vi "executeBuildSpecs.vi"() -> ()   [LabVIEW 2023]
doc: "Execute Build Specs G-CLI.vi\n----------------------------------------------\nThis VI is used to build the lvlibp from the build specifications.\n\nInputs:\n---------------------\n\n\nOutputs:\n---------------------\n\n\n----------------------------------------------\n1/27/2021 nina\nZühlke Engineering AG\nCH-8952 Schlieren\nwww.zuehlke.com"
uses:
  <vilib>/AppBuilder/AB_API_Simple/Get Build Specification Version (path).vi
  <vilib>/Wiresmith Technology/G CLI/CLI Class/CLI.lvclass
  <vilib>/AppBuilder/AB_API_Simple/NI_App_Builder_API.lvlib
panel:
  out "error out":errorcluster
  out "Build Specification Names":string[](array[string])
  # "Locals"
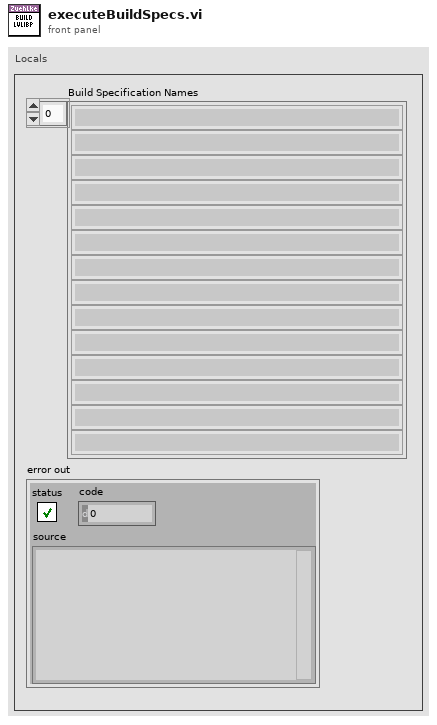
[diagram p1: front panel]
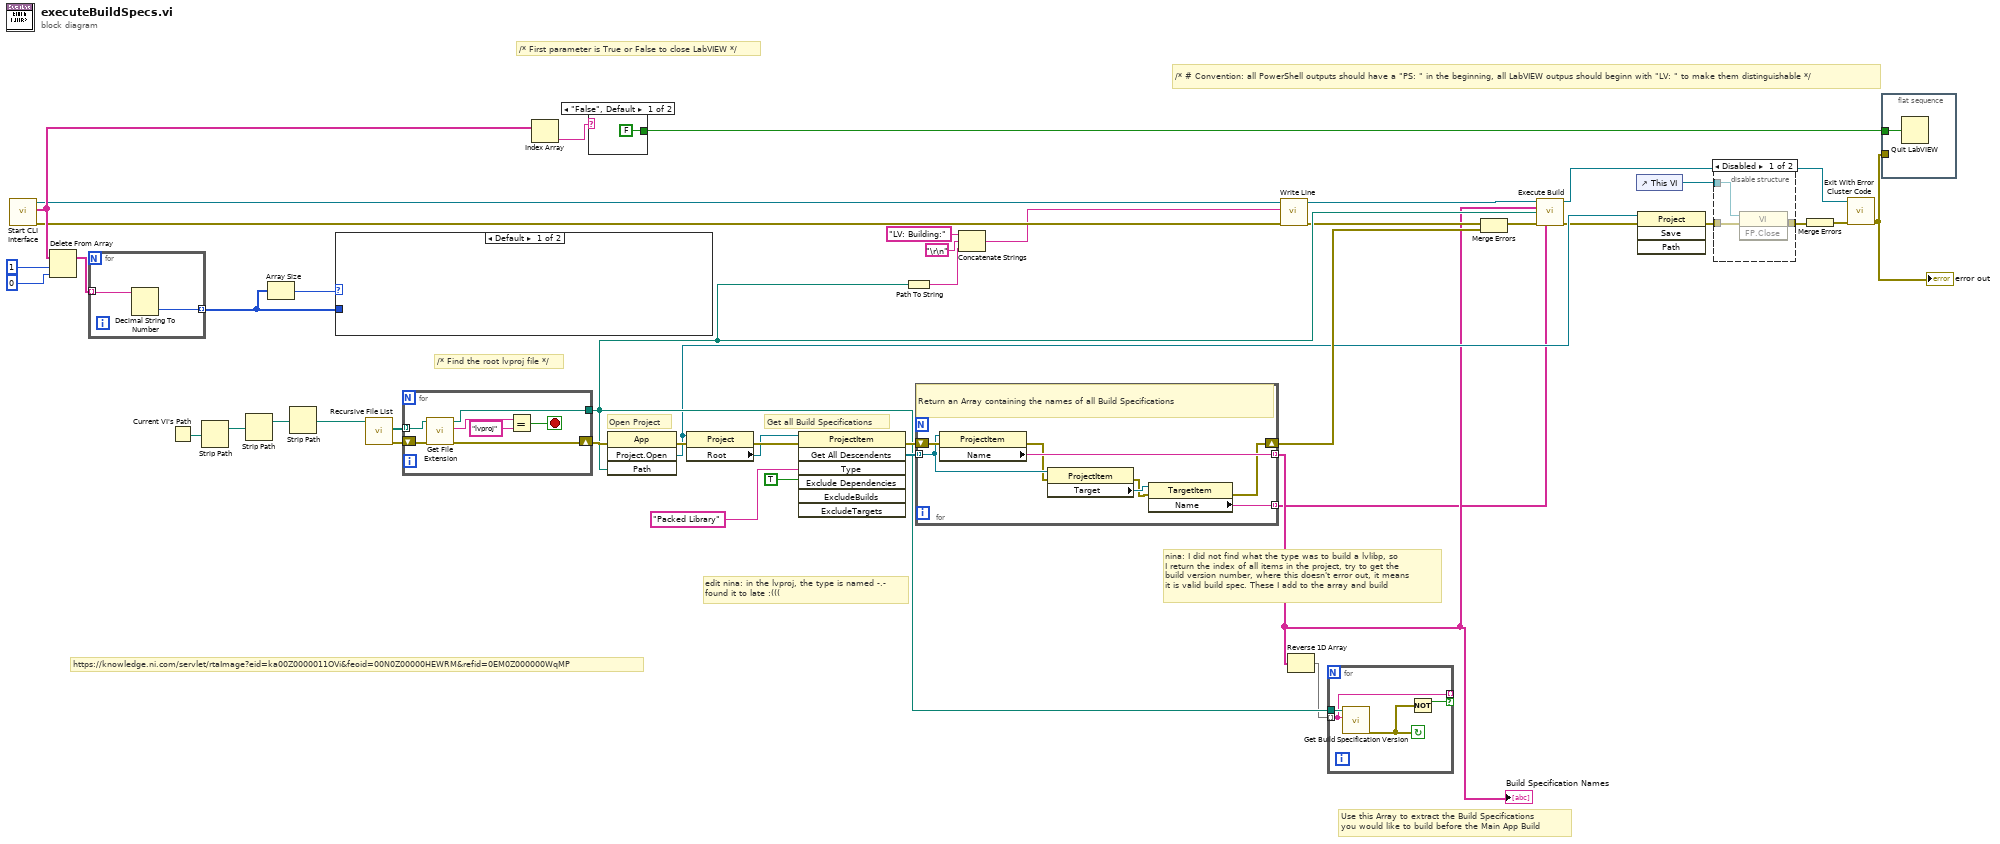
[diagram p0: block diagram]
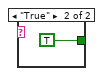
[diagram p2: hidden frame]
diagram:
  # "/* # Convention: all PowerShell outputs should have a \"PS: \" in the beginning, all LabVIEW outpus should beginn with \"LV: \" to make them distinguishable */"
  # "edit nina: in the lvproj, the type is named -.-\nfound it to late :((("
  # "nina: I did not find what the type was to build a lvlibp, so\nI return the index of all items in the project, try to get the \nbuild version number, where this doesn't error out, it means\nit is valid build spec. These I add to the array and build"
  # "/* First parameter is True or False to close LabVIEW */"
  # "Use this Array to extract the Build Specifications \nyou would like to build before the Main App Build"
  # "Get all Build Specifications"
  # "Open Project"
  # "https://knowledge.ni.com/servlet/rtaImage?eid=ka00Z0000011OVi&feoid=00N0Z00000HEWRM&refid=0EM0Z000000WqMP"
  # "/* Find the root lvproj file */"
  n1 = call <vilib>:"Start CLI Interface.vi"() -> ("error out"=w22:errorcluster, "Custom Parameters"=w28:string[], "CLI out"=w24:refnum<class "CLI.lvclass">)  [unwired: 8 in, 1 out]
  n2 = Delete From Array(array=w28, length=1, index=0) -> (array with subset deleted=w25:string[])  [unwired: 1 out]
  n3 = for {
    tunnel: w25 -> [w46] mode=indexing
    tunnel: [w45] -> w31 mode=indexing
    n4 = Decimal String To Number(string=w46) -> (number=w45:i32)  [unwired: 2 in, 1 out]
  }
  n5 = Current VI's Path() -> (path=w44:path)
  n6 = Strip Path(path=w44) -> (stripped path=w41:path)  [unwired: 1 out]
  n7 = Strip Path(path=w41) -> (stripped path=w18:path)  [unwired: 1 out]
  n8 = Array Size(array=w31) -> (size(s)=w32:i32)
  n9 = Strip Path(path=w18) -> (stripped path=w1:path)  [unwired: 1 out]
  n10 = case shown="Default" w32 {
    tunnel: w31 -> [_ _]
    frame Default {
    }
    frame 0 {
      # "If array is empty and no build specs have been defined, revert to building the first EXE"
    }
  }
  n11 = call <vilib>:"Recursive File List.vi"("Folder Path"=w1) -> ("error out"=w42:errorcluster, "All Files in Dir"=w43:path[])  [unwired: 6 in, 3 out]
  n12 = for {
    tunnel: w43 -> [w53] mode=indexing
    tunnel: [w49] -> w17
    shift-right: [w47] -> w34
    shift-left: w42 -> [w48]
    stop <- w50 stop-if-true
    n13 = call <vilib>:"Get File Extension.vi"("error in (no error)"=w48, "file"=w53) -> ("error out"=w47:errorcluster, "lowercase file extension"=w52:string, "dup file"=w49:path)  [unwired: 5 in, 2 out]
    n14 = Equal?(x=w52, y="lvproj") -> (x = y?=w50:bool)
  }
  n15 = Index Array(array=w28) -> (element=w30:string)  [unwired: 1 in]
  n16 = case shown="\"False\", Default" w30 {
    tunnel: [FALSE TRUE] -> w29
    frame "False", Default {
    }
    frame "True" {
    }
  }
  n17 = invoke class="App" method="Project.Open"(error in=w34, "Path"=w17) -> (error out=w37:errorcluster, "Project:Open"=w8:refnum<vi>)  [unwired: 2 in, 2 out]
  n18 = property class="Project"(reference=w8, error in=w37) -> (error out=w39:errorcluster, "Root"=w38:refnum<vi>)  [unwired: 1 out]
  n19 = invoke class="ProjectItem" method="Get All Descendents"(reference=w38, error in=w39, "Type"="Packed Library", "Exclude Dependencies"=TRUE ("ExcludeDependencies")) -> (error out=w35:errorcluster, "All Descendents"=w36:refnum<vi>[])  [unwired: 3 in, 5 out]
  n20 = Path To String(path=w17) -> (string=w19:string)
  n21 = for {
    tunnel: w36 -> [w61] mode=indexing
    tunnel: [w63] -> w3 mode=indexing
    shift-right: [w57] -> w11
    shift-left: w35 -> [w62]
    tunnel: [w56] -> w2 mode=indexing
    # "Return an Array containing the names of all Build Specifications"
    n22 = property class="ProjectItem"(reference=w61, error in=w62) -> (error out=w59:errorcluster, "Name"=w63:string)  [unwired: 1 out]
    n23 = property class="ProjectItem"(reference=w61, error in=w59) -> (error out=w58:errorcluster, "Target"=w60:refnum<vi>)  [unwired: 1 out]
    n24 = property class="TargetItem"(reference=w60, error in=w58) -> (error out=w57:errorcluster, "Name"=w56:string)  [unwired: 1 out]
  }
  "Build Specification Names" <- w3
  n25 = Concatenate Strings("LV: Building:" ("string"), "\r\n", w19) -> (w9:string)
  n26 = call <vilib>:"Write Line.vi"("error in (no error)"=w22, "Text to Write"=w9, "CLI in"=w24) -> ("error out"=w13:errorcluster, "CLI out"=w23:refnum<class "CLI.lvclass">)  [unwired: 7 in]
  n27 = Reverse 1D Array(array=w3) -> (reversed array=w16:string[])
  n28 = for {
    tunnel: w17 -> [w67]
    tunnel: w16 -> [w66] mode=indexing
    tunnel: [w66] -> _ mode=indexing if=w65
    stop <- w64 continue-if-true
    n29 = call-poly <vilib>:"Get Build Specification Version.vi"("Name of build specification"=w66, "Path to project"=w67) -> ("error out"=w64:errorcluster)  [unwired: 8 in, 1 out]
    n30 = Not(x=w64) -> (.not. x?=w65:bool)
  }
  n31 = Merge Errors(w13, w11) -> (w12:errorcluster)
  n32 = call "Execute Build.vi"("CLI in"=w23, "All Build Specs"=w3, "Proj Path"=w17, "error in (no error)"=w12, "Targets"=w2) -> ("CLI out"=w14:refnum<class "CLI.lvclass">, "error out"=w7:errorcluster)  [unwired: 8 in, 1 out]
  n33 = control-ref of="This VI"() -> (w5:refnum<vi>)
  n34 = invoke class="Project" method="Save"(reference=w8, error in=w7) -> (error out=w4:errorcluster)  [unwired: 2 in, 3 out]
  n35 = disable-structure shown="Disabled" {
    disable-tunnel: [w70 w71] -> w6
    disable-tunnel: w5 -> [w69 _]
    disable-tunnel: w4 -> [w68 w71]
    frame Disabled {
      n36 = invoke class="VI" method="FP.Close"(reference=w69, error in=w68) -> (error out=w70:errorcluster)  [unwired: 1 in, 2 out]
    }
    frame Enabled {
    }
  }
  n37 = Merge Errors(w6) -> (w33:errorcluster)
  n38 = call <vilib>:"Exit With Error Cluster Code.vi"("error in (no error)"=w33, "CLI in"=w14) -> ("error out"=w10:errorcluster)  [unwired: 9 in]
  "error out" <- w10
  n39 = flat-sequence {
    tunnel: w29 -> [w72]
    tunnel: w10 -> [_]
    frame #0 {
      n40 = Quit LabVIEW(quit? (T)=w72) -> ()
    }
  }
